vi "GPIBReadCurr.vi"(1 "address string":string="7") -> (0 "current":dbl format="%^.2e")   [LabVIEW 2015]
panel:
  out "error out":errorcluster
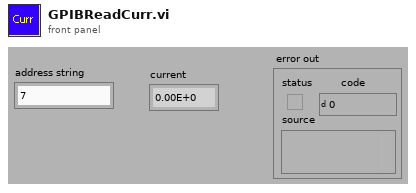
[diagram p1: front panel]
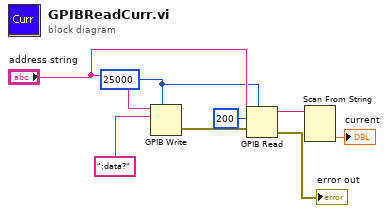
[diagram p0: block diagram]
diagram:
  w1 = 25000 ("timeout ms (488.2 global)")
  n1 = GPIB Write(0:"address string", 1:":data?" ("data"), 4:w1) -> (6:w7:errorcluster)  [unwired: 2 in, 1 out]
  n2 = GPIB Read(0:"address string", 1:200 ("byte count"), 3:w7, 4:w1) -> (5:w4:string, 7:→"error out":errorcluster)  [unwired: 1 in, 1 out]
  n3 = Scan From String(input string=w4) -> (output 1=→"current":dbl)  [unwired: 4 in, 3 out]
